vi "Pasco Auton Pack.vi"(0 "Iterations":i32, 1 "Left Drive":dbl, 2 "Right Drive":dbl, 3 "RAMP ACT":dbl, 4 "Conveyor":dbl, 5 "Harvestor":dbl, 6 "Auton Array":dbl[][](array[numeric]), 7 "Turret":dbl, 9 "Shooter":dbl) -> (14 "Iteration Output":i32, 16 "output array":dbl[][](array[numeric]))   [LabVIEW 2011]
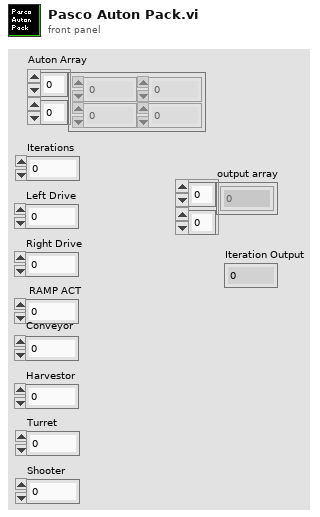
[diagram p1: front panel]
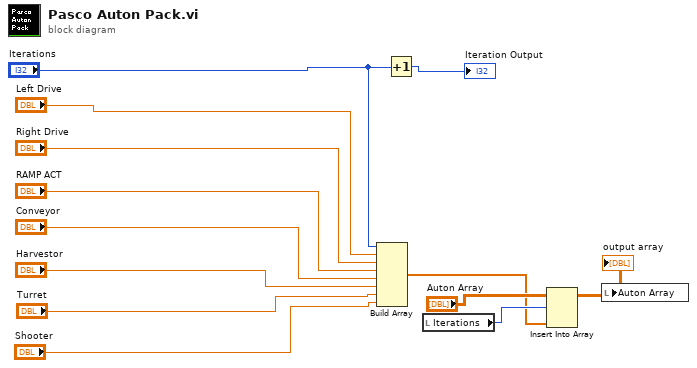
[diagram p0: block diagram]
diagram:
  n1 = Build Array("Iterations", "Left Drive", "Right Drive", "RAMP ACT", "Conveyor", "Harvestor", "Turret", "Shooter") -> (w1:dbl[])
  n2 = Increment(x="Iterations") -> (x+1=→"Iteration Output":i32)
  n3 = local read "Iterations"() -> (w10:i32)
  n4 = Insert Into Array(array="Auton Array", index (row)=w10, new element=w1) -> (w11:dbl[][])  [unwired: 1 in]
  "output array" <- w11
  n5 = local write "Auton Array"(w11) -> ()
